vi "FFT滤波.vi"(0 "low cutoff freq: fl":dbl=0.12500000000000006 caption="低截止频率:fl" format="%0.4f", 2 "high cutoff freq: fh":dbl=0.45000000000000007 caption="高截止频率:fh" format="%0.2f", 3 "时域波形图":waveform(dbl)[](graph), 4 "order":i32=2 caption="阶数", 5 "filter type":T1 caption="滤波器类型", 6 "采样频率":dbl=1.0 caption="采样频率:fs" format="%0.2f") -> (1 "时域波形图 2":waveform(dbl)[](graph))   [LabVIEW 2014]
uses:
  <vilib>/Analysis/3filter.llb/Filter Passband Type.ctl
  <vilib>/Analysis/2dsp.llb/Real FFT.vi
  <vilib>/Analysis/2dsp.llb/Inverse Real FFT.vi
  <vilib>/Analysis/3filter.llb/Butterworth Filter (CDB).vi
  <vilib>/express/express analysis/Spectral/Block/exnSpectralBlock spectral measurements peak poly.vi
  <vilib>/express/express analysis/Spectral/Block/exnSpectralBlock spectral measurements peak WFM.vi
  <vilib>/express/express analysis/Spectral/XNode/ExpressSpectralMeasurementsBlockNode.xnode
  <vilib>/Analysis/NI_AALPro.lvlib
  <vilib>/Analysis/NI_AALBase.lvlib
panel:
  out "时域波形图 3":cluster{"f0":dbl, "df":dbl, "magnitude":dbl[]}(graph)
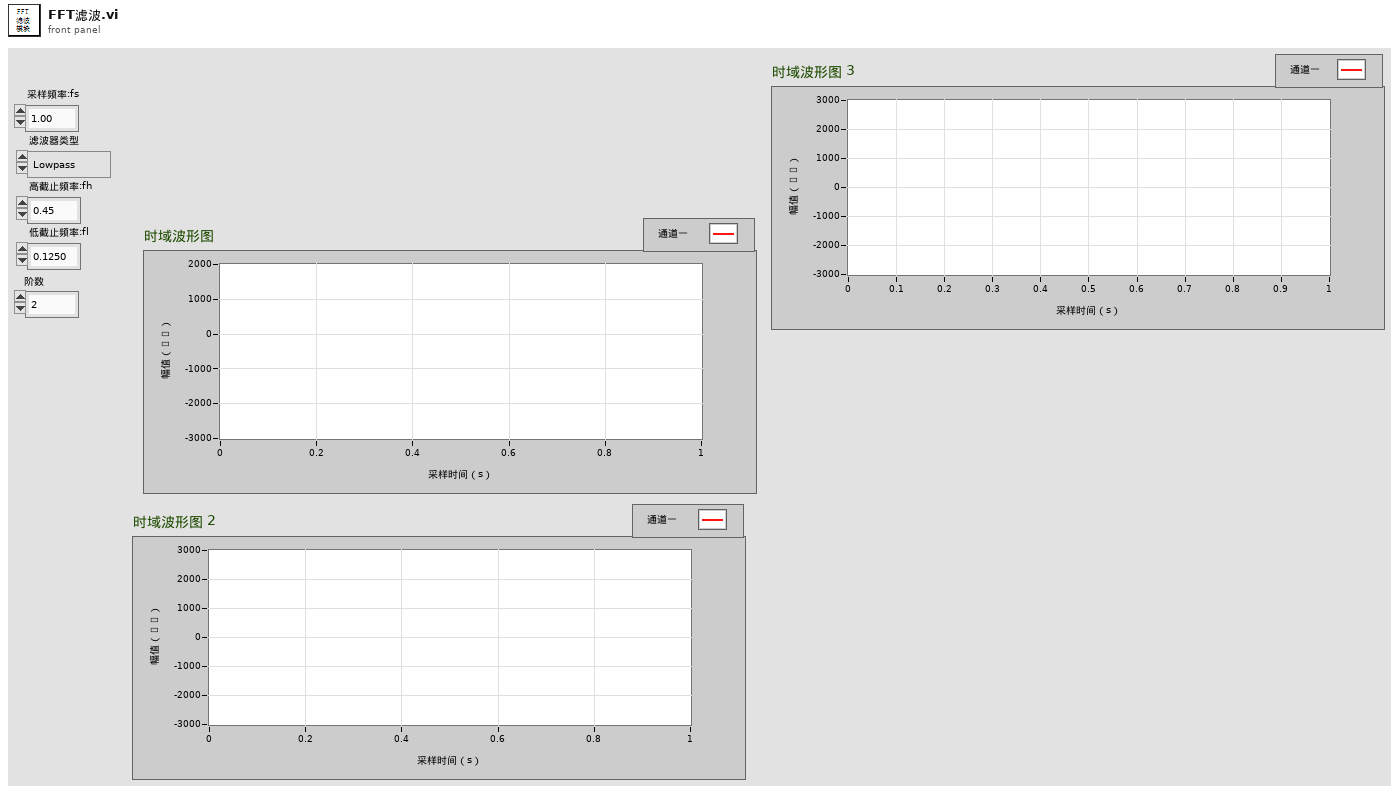
[diagram p1: front panel]
types:
  T1 = typedef "NI_AALBase.lvlib/Filter Passband Type.ctl" = enum32{"Lowpass", "Highpass", "Bandpass", "Bandstop"}
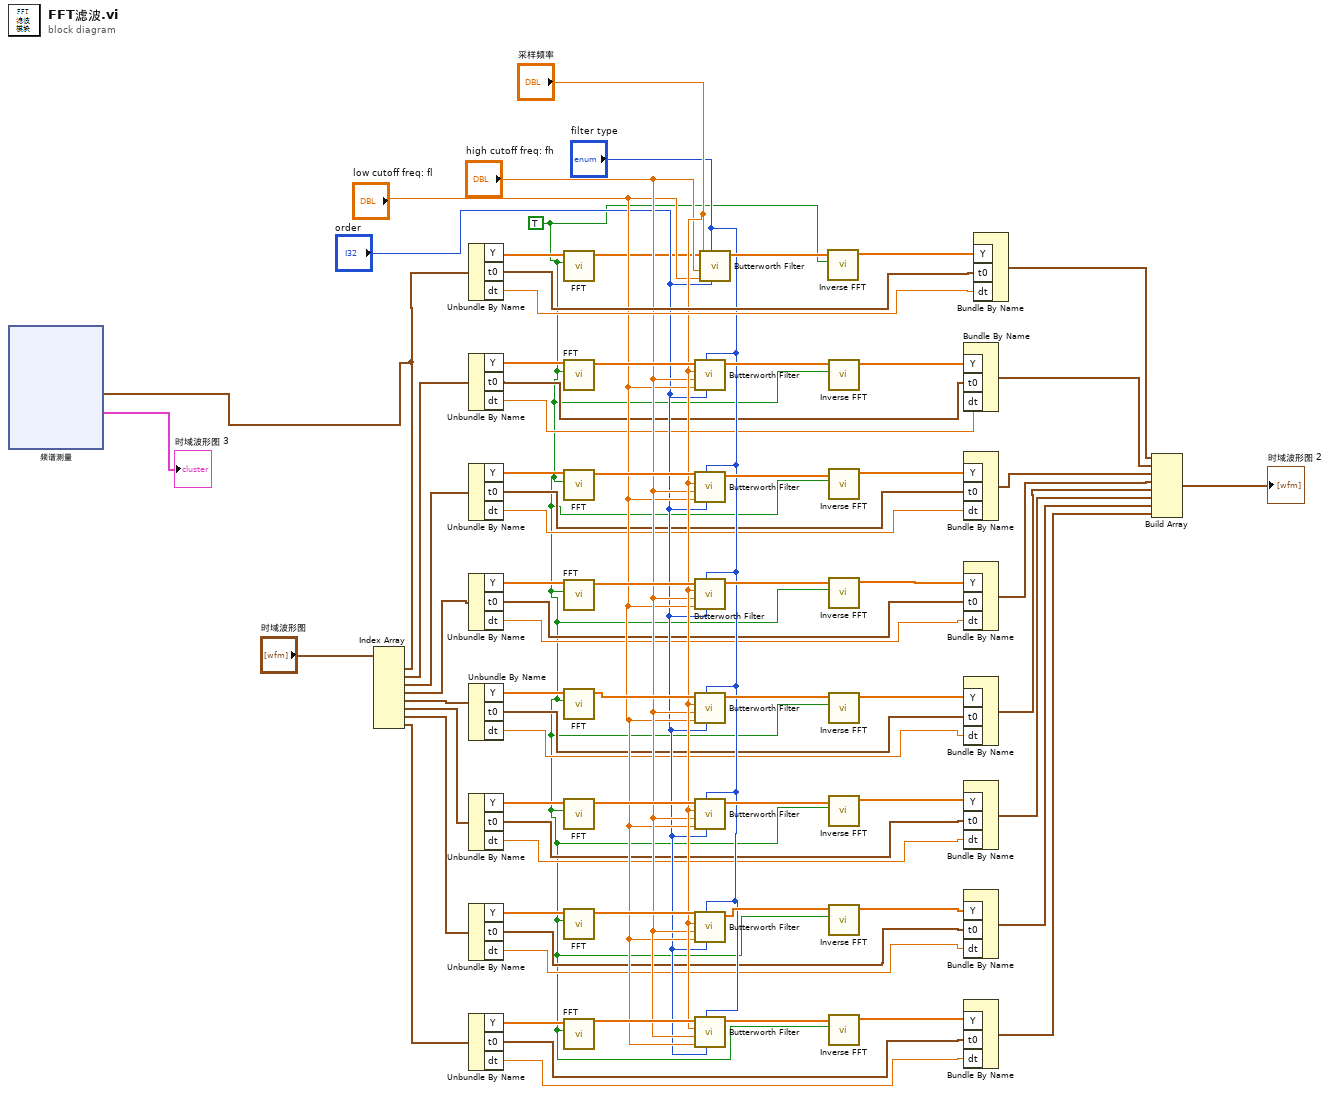
[diagram p0: block diagram]
diagram:
  w4 = TRUE
  n1 = Index Array(array="时域波形图") -> (element #1=w3:waveform(dbl), element #2=w72:waveform(dbl), element #3=w71:waveform(dbl), element #4=w70:waveform(dbl), element #5=w69:waveform(dbl), element #6=w68:waveform(dbl), element #7=w67:waveform(dbl), element #8=w66:waveform(dbl))  [unwired: 8 in]
  n2 = xnode "频谱测量"("信号"=w3) -> ("FFT - （峰值）"=→"时域波形图 3":cluster{"f0":dbl, "df":dbl, "magnitude":dbl[]})  [unwired: 1 in, 2 out]
  n3 = Unbundle By Name(w3) -> ("Y"=w65:dbl[], "t0"=w57:timestamp, "dt"=w56:dbl)
  n4 = Unbundle By Name(w72) -> ("Y"=w63:dbl[], "t0"=w27:timestamp, "dt"=w26:dbl)
  n5 = Unbundle By Name(w71) -> ("Y"=w62:dbl[], "t0"=w25:timestamp, "dt"=w24:dbl)
  n6 = Unbundle By Name(w70) -> ("Y"=w61:dbl[], "t0"=w23:timestamp, "dt"=w22:dbl)
  n7 = Unbundle By Name(w69) -> ("Y"=w60:dbl[], "t0"=w21:timestamp, "dt"=w20:dbl)
  n8 = Unbundle By Name(w68) -> ("Y"=w41:dbl[], "t0"=w19:timestamp, "dt"=w18:dbl)
  n9 = Unbundle By Name(w67) -> ("Y"=w40:dbl[], "t0"=w17:timestamp, "dt"=w16:dbl)
  n10 = Unbundle By Name(w66) -> ("Y"=w64:dbl[], "t0"=w15:timestamp, "dt"=w14:dbl)
  n11 = call-poly <vilib>:"FFT.vi"("shift?"=w4, "X"=w65) -> ("FFT {X}"=w1:cdb[])  [unwired: 8 in, 1 out]
  n12 = call-poly <vilib>:"FFT.vi"("shift?"=w4, "X"=w63) -> ("FFT {X}"=w55:cdb[])  [unwired: 8 in, 1 out]
  n13 = call-poly <vilib>:"FFT.vi"("shift?"=w4, "X"=w62) -> ("FFT {X}"=w50:cdb[])  [unwired: 8 in, 1 out]
  n14 = call-poly <vilib>:"FFT.vi"("shift?"=w4, "X"=w61) -> ("FFT {X}"=w47:cdb[])  [unwired: 8 in, 1 out]
  n15 = call-poly <vilib>:"FFT.vi"("shift?"=w4, "X"=w60) -> ("FFT {X}"=w44:cdb[])  [unwired: 8 in, 1 out]
  n16 = call-poly <vilib>:"FFT.vi"("shift?"=w4, "X"=w41) -> ("FFT {X}"=w38:cdb[])  [unwired: 8 in, 1 out]
  n17 = call-poly <vilib>:"FFT.vi"("shift?"=w4, "X"=w40) -> ("FFT {X}"=w39:cdb[])  [unwired: 8 in, 1 out]
  n18 = call-poly <vilib>:"FFT.vi"("shift?"=w4, "X"=w64) -> ("FFT {X}"=w52:cdb[])  [unwired: 8 in, 1 out]
  n19 = call-poly <vilib>:"Butterworth Filter.vi"("order"="order", "filter type"="filter type", "low cutoff freq: fl"="low cutoff freq: fl", "high cutoff freq: fh"="high cutoff freq: fh", "sampling freq: fs"="采样频率", "X"=w55) -> ("Filtered X"=w54:cdb[])  [unwired: 2 in, 1 out]
  n20 = call-poly <vilib>:"Butterworth Filter.vi"("order"="order", "filter type"="filter type", "low cutoff freq: fl"="low cutoff freq: fl", "high cutoff freq: fh"="high cutoff freq: fh", "sampling freq: fs"="采样频率", "X"=w50) -> ("Filtered X"=w49:cdb[])  [unwired: 2 in, 1 out]
  n21 = call-poly <vilib>:"Butterworth Filter.vi"("order"="order", "filter type"="filter type", "low cutoff freq: fl"="low cutoff freq: fl", "high cutoff freq: fh"="high cutoff freq: fh", "sampling freq: fs"="采样频率", "X"=w47) -> ("Filtered X"=w46:cdb[])  [unwired: 2 in, 1 out]
  n22 = call-poly <vilib>:"Butterworth Filter.vi"("order"="order", "filter type"="filter type", "low cutoff freq: fl"="low cutoff freq: fl", "high cutoff freq: fh"="high cutoff freq: fh", "sampling freq: fs"="采样频率", "X"=w44) -> ("Filtered X"=w43:cdb[])  [unwired: 2 in, 1 out]
  n23 = call-poly <vilib>:"Butterworth Filter.vi"("order"="order", "filter type"="filter type", "low cutoff freq: fl"="low cutoff freq: fl", "high cutoff freq: fh"="high cutoff freq: fh", "sampling freq: fs"="采样频率", "X"=w38) -> ("Filtered X"=w37:cdb[])  [unwired: 2 in, 1 out]
  n24 = call-poly <vilib>:"Butterworth Filter.vi"("order"="order", "filter type"="filter type", "low cutoff freq: fl"="low cutoff freq: fl", "high cutoff freq: fh"="high cutoff freq: fh", "sampling freq: fs"="采样频率", "X"=w39) -> ("Filtered X"=w35:cdb[])  [unwired: 2 in, 1 out]
  n25 = call-poly <vilib>:"Butterworth Filter.vi"("order"="order", "filter type"="filter type", "low cutoff freq: fl"="low cutoff freq: fl", "high cutoff freq: fh"="high cutoff freq: fh", "sampling freq: fs"="采样频率", "X"=w52) -> ("Filtered X"=w51:cdb[])  [unwired: 2 in, 1 out]
  n26 = call-poly <vilib>:"Butterworth Filter.vi"("order"="order", "filter type"="filter type", "low cutoff freq: fl"="low cutoff freq: fl", "high cutoff freq: fh"="high cutoff freq: fh", "sampling freq: fs"="采样频率", "X"=w1) -> ("Filtered X"=w59:cdb[])  [unwired: 2 in, 1 out]
  n27 = call-poly <vilib>:"Inverse FFT.vi"("shift?"=w4, "FFT {X}"=w59) -> ("X"=w58:dbl[])  [unwired: 8 in, 1 out]
  n28 = call-poly <vilib>:"Inverse FFT.vi"("shift?"=w4, "FFT {X}"=w54) -> ("X"=w53:dbl[])  [unwired: 8 in, 1 out]
  n29 = call-poly <vilib>:"Inverse FFT.vi"("shift?"=w4, "FFT {X}"=w49) -> ("X"=w48:dbl[])  [unwired: 8 in, 1 out]
  n30 = call-poly <vilib>:"Inverse FFT.vi"("shift?"=w4, "FFT {X}"=w46) -> ("X"=w45:dbl[])  [unwired: 8 in, 1 out]
  n31 = call-poly <vilib>:"Inverse FFT.vi"("shift?"=w4, "FFT {X}"=w43) -> ("X"=w42:dbl[])  [unwired: 8 in, 1 out]
  n32 = call-poly <vilib>:"Inverse FFT.vi"("shift?"=w4, "FFT {X}"=w37) -> ("X"=w36:dbl[])  [unwired: 8 in, 1 out]
  n33 = call-poly <vilib>:"Inverse FFT.vi"("shift?"=w4, "FFT {X}"=w35) -> ("X"=w34:dbl[])  [unwired: 8 in, 1 out]
  n34 = call-poly <vilib>:"Inverse FFT.vi"("shift?"=w4, "FFT {X}"=w51) -> ("X"=w33:dbl[])  [unwired: 8 in, 1 out]
  n35 = Bundle By Name("Y"=w53, "t0"=w27, "dt"=w26) -> (w12:waveform(dbl))  [unwired: 1 in]
  n36 = Bundle By Name("Y"=w48, "t0"=w25, "dt"=w24) -> (w11:waveform(dbl))  [unwired: 1 in]
  n37 = Bundle By Name("Y"=w45, "t0"=w23, "dt"=w22) -> (w10:waveform(dbl))  [unwired: 1 in]
  n38 = Bundle By Name("Y"=w42, "t0"=w21, "dt"=w20) -> (w9:waveform(dbl))  [unwired: 1 in]
  n39 = Bundle By Name("Y"=w36, "t0"=w19, "dt"=w18) -> (w8:waveform(dbl))  [unwired: 1 in]
  n40 = Bundle By Name("Y"=w34, "t0"=w17, "dt"=w16) -> (w7:waveform(dbl))  [unwired: 1 in]
  n41 = Bundle By Name("Y"=w33, "t0"=w15, "dt"=w14) -> (w6:waveform(dbl))  [unwired: 1 in]
  n42 = Bundle By Name("Y"=w58, "t0"=w57, "dt"=w56) -> (w13:waveform(dbl))  [unwired: 1 in]
  n43 = Build Array(w13, w12, w11, w10, w9, w8, w7, w6) -> (→"时域波形图 2":waveform(dbl)[])
